vi "Action.vi"(7 "Assert Message":T1, 8 "error in (no error)":errorcluster, 11 "Abort Application in":refnum<class "Abort Application.lvclass">) -> (0 "error out":errorcluster)   [LabVIEW 2016, in "Assert API Components.lvlib" / "Log Assert Core.lvlib" / "Abort Application.lvclass"]
doc: "Dynamic dispatch vi which is triggered when an assert fails and the failure action is set to Abort.\nAborts the VI and displays a dialog box with details of the failure"
uses:
  Abort Application.lvclass
  Message Data.ctl
  Failure Actions.ctl
  VI References.ctl
  Assert API Components.lvlib
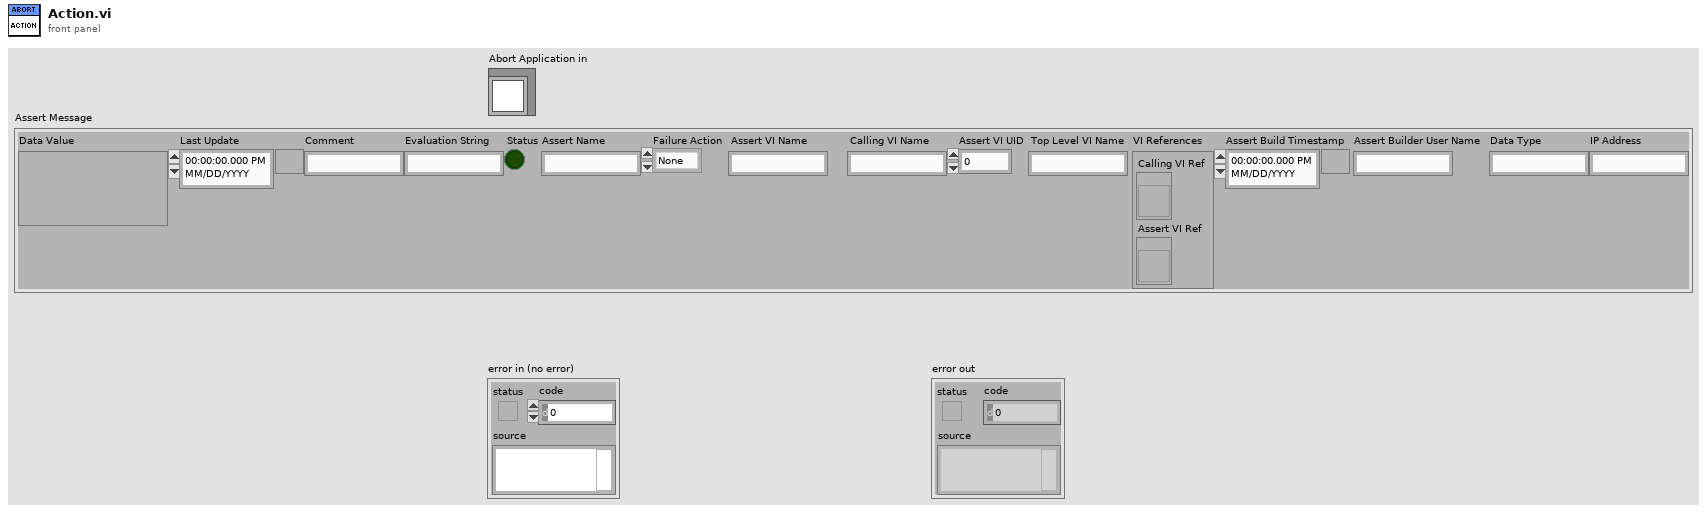
[diagram p1: front panel]
types:
  T1 = typedef "Assert API Components.lvlib/Message Data.ctl" = cluster{"Data Value":variant, "Last Update":timestamp, "Comment":string, "Evaluation String":string, "Status":bool, "Assert Name":string, "Failure Action":T2, "Assert VI Name":string, "Calling VI Name":string, "Assert VI UID":i32, "Top Level VI Name":string, "VI References":T3, "Assert Build Timestamp":timestamp, "Assert Builder User Name":string, "Data Type":string, "IP Address":string}
  T2 = typedef "Assert API Components.lvlib/Failure Actions.ctl" = enum16{"None", "Log To File", "Pause Execution", "Abort Execution"}
  T3 = typedef "Assert API Components.lvlib/VI References.ctl" = cluster{"Calling VI Ref":refnum<vi>, "Assert VI Ref":refnum<vi>}
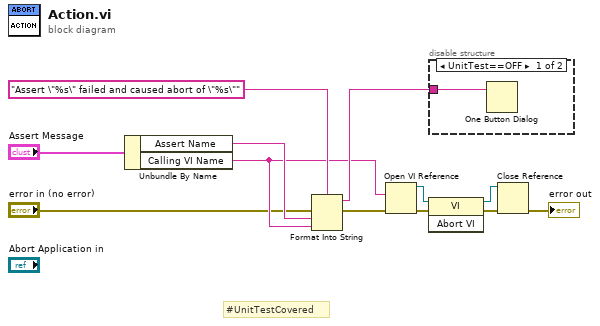
[diagram p0: block diagram]
diagram:
  # "#UnitTestCovered"
  n1 = Unbundle By Name("Assert Message") -> ("Assert Name"=w5:string, "Calling VI Name"=w4:string)
  n2 = Format Into String(format string="Assert \"%s\" failed and caused abort of \"%s\"", error in="error in (no error)", w5, w4) -> (resulting string=w8:string, error out=w2:errorcluster)  [unwired: 1 in]
  n3 = Open VI Reference(vi path=w4, error in (no error)=w2) -> (vi reference=w12:refnum<vi>, error out=w11:errorcluster)  [unwired: 4 in]
  n4 = invoke class="VI" method="Abort VI"(reference=w12, error in=w11) -> (reference out=w10:refnum<vi>, error out=w9:errorcluster)  [unwired: 1 in, 1 out]
  n5 = disable-structure shown="UnitTest==OFF" {
    disable-tunnel: w8 -> [w13 _]
    frame condition #0 (active) {
      n6 = One Button Dialog(message=w13) -> ()  [unwired: 1 in, 1 out]
    }
    frame condition #1 {
    }
  }
  n7 = Close Reference(reference=w10, error in (no error)=w9) -> (error out=→"error out":errorcluster)
